vi "Icai 105.vi"() -> ()   [LabVIEW 2010]
uses:
  <vilib>/Utility/error.llb/DialogType.ctl
  <vilib>/DAQmx/write.llb/DAQmx Write (Analog DBL 1Chan 1Samp).vi
  <vilib>/DAQmx/create/channels.llb/DAQmx Create Channel (AO-Voltage-Basic).vi
  <vilib>/daqmx/miscellaneous.llb/DAQmx Fill In Error Info.vi
  <vilib>/Waveform/WDTOps.llb/WDT Append Waveforms DBL.vi
  <vilib>/measure/NI_MABase.lvlib
panel:
  out "Mod":dbl=118572.0
  out "Numeric 2":dbl=3900000.0 format="%#_7g"
  out "Numeric":dbl=3900000.0 format="%#_7g"
  in  "CAI/ICAI":bool=TRUE
  in  "DC 2":ext=3710.75 format="%.2f"
  out "?":dbl=579698.7113293351 format="%#_6f"
  in  "Fs":dbl=1000000.0
  out "#s":dbl=39524.02451426849
  in  "Time int":i32=32000
  in  "Sensitivity":u16(ring)=21 items=["2 nV/fA", "5 nV/fA", "10 nV/fA", "20 nV/fA", "50 nV/fA", "100 nV/fA", "200 nV/fA", "500 nV/fA", "1 uV/pA", "2 uV/pA", "5 uV/pA", "10 uV/pA", "20 uV/pA", "50 uV/pA", "100 uV/pA", "200 uV/pA", "500 uV/pA", "1 mV/nA", "2 mV/nA", "5 mV/nA", "10 mV/nA", "20 mV/nA", "50 mV/nA", "100 mV/nA", "200 mV/nA", "500 mV/nA", "1 V/uA"]
  in  "Detection Bandwidth":u16(ring)=7 items=["25 kHz", "8.33 kHz", "2.50 kHz", "833 Hz", "250 Hz", "83.3 Hz", "25 Hz", "8.33 Hz", "2.50 Hz", "0.833 Hz", "0.250 Hz", "0.0833 Hz", "0.025 Hz"]
  in  "SR 830 GPIB Address":i32=8
  in  "Freq 2":dbl=6401.17 format="%_7g"
  out "Iterat #":dbl=10.0
  in  "Iteration":dbl=10.0
  in  "stop 2":bool
  in  "pulse":bool=TRUE
  in  "Start":ext=0.2
  out "?":waveform(dbl)[](graph)=[{"t0"=timestamp(0 s since 1904-01-01), "dt"=1e-06, "Y"=array[3900000 elements]}, {"t0"=timestamp(0 s since 1904-01-01), "dt"=1e-06, "Y"=array[3900000 elements]}]
  in  "amplitude 2":dbl=0.25 format="%0.2p"
  in  "?":T1(ring)=enum."Triangle Wave"
  in  "phase 2":dbl format="%.2p"
  in  "Offset 2":dbl=-0.0 format="%#_6p"
  in  "frequency 4":dbl=100.0 format="%0.2p"
  in  "sampling info 4":cluster{"Fs":dbl, "#s":dbl}={"Fs"=1000000.0, "#s"=2499.0} {"Fs" format="%.2p"}
  in  "?":T1(ring)=enum."Triangle Wave"
  in  "offset 4":dbl=-1.0 format="%0.2p"
  in  "phase 4":dbl=90.0 format="%.2p"
  in  "amplitude 4":dbl=1.0 format="%0.2p"
  in  "frequency 1":dbl=100.0 format="%0.2p"
  in  "amplitude 1":dbl=1.0 format="%0.2p"
  in  "sampling info 1":cluster{"Fs":dbl, "#s":dbl}={"Fs"=1000000.0, "#s"=2500.0} {"Fs" format="%.2p"}
  in  "?":T1(ring)=enum."Triangle Wave"
  in  "phase 1":dbl=-90.0 format="%.2p"
  in  "Offset 1":dbl format="%#_6p"
  in  "iterat":dbl=2.0
  out "CW":dbl=123571.0
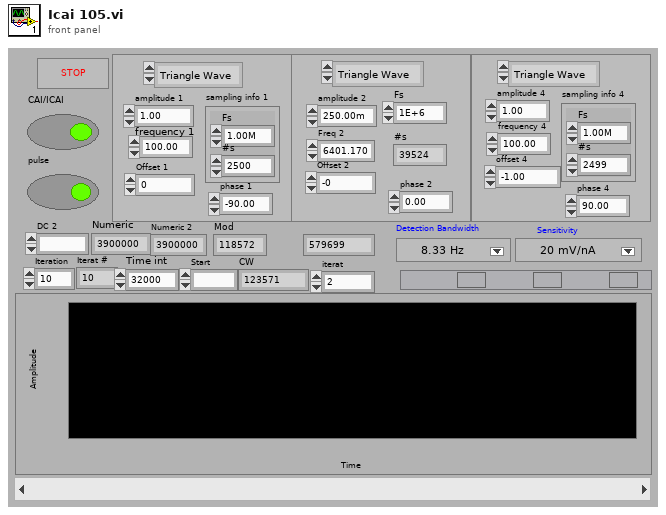
[diagram p1: front panel]
types:
  T1 = enum16{"Sine Wave", "Triangle Wave", "Square Wave", "Sawtooth Wave"}
  T2 = typedef "DialogType.ctl" = u16
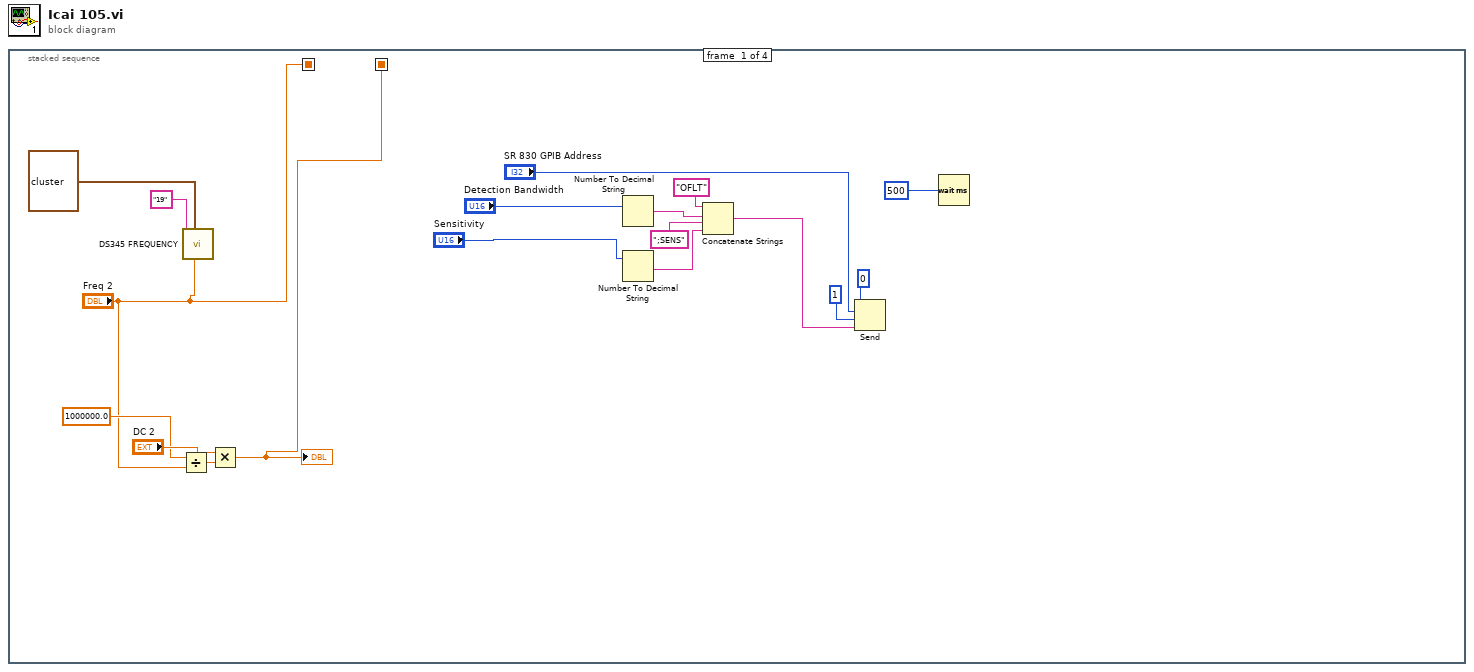
[diagram p0: block diagram]
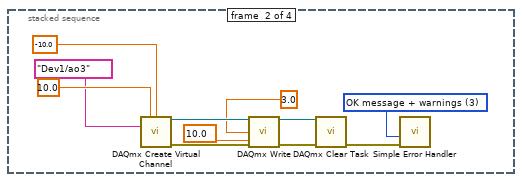
[diagram p2: hidden frame]
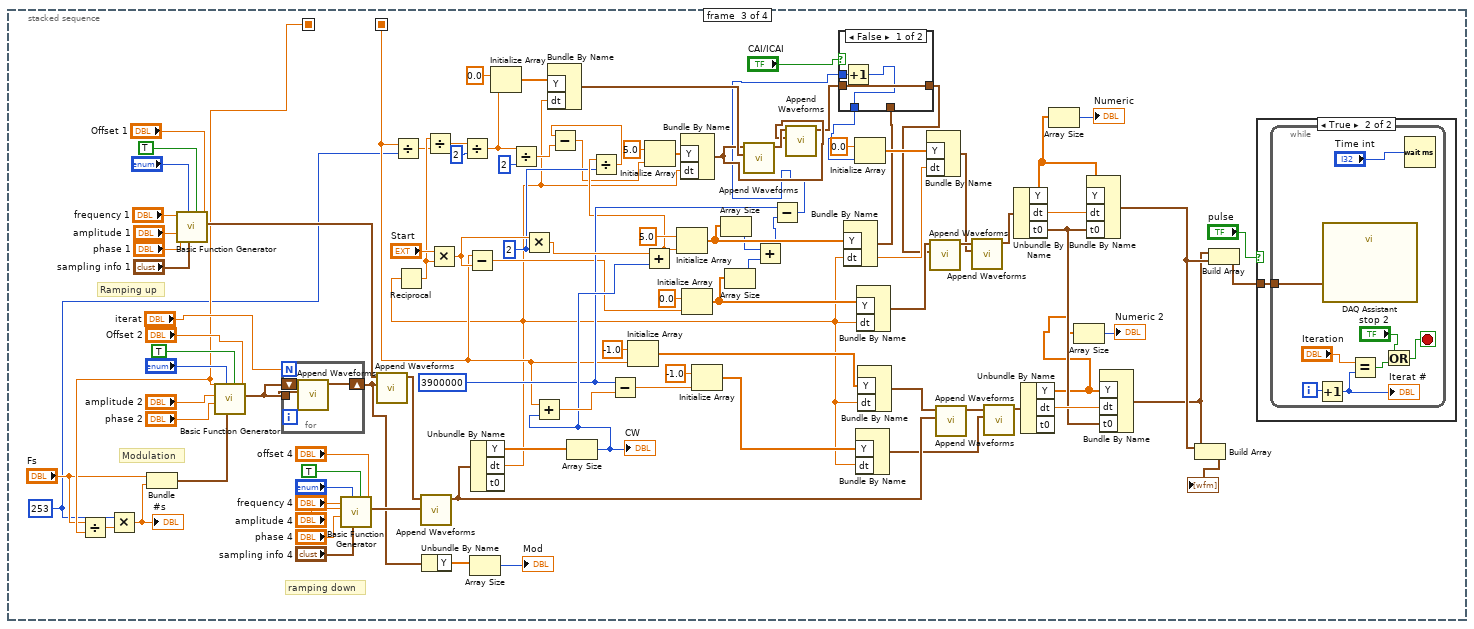
[diagram p3: hidden frame]
diagram:
  n1 = stacked-sequence {
    seq-local: ["Freq 2" _ _ _] -> [_ _ w68 _]
    seq-local: [w2 _ _ _] -> [_ _ w53 _]
    frame #0 {
      n2 = Divide(x=1000000.0 ("Fs 2"), y="Freq 2") -> (x/y=w5:dbl)
      n3 = call "DS345 FREQUENCY.vi"("GPIB address"="19", "amplitude (0 Vrms:0)"=cluster{ext, i32} {0.02, 0} ("Driving amplitude (0 Vrms:0)"), "frequency"="Freq 2") -> ()  [unwired: 5 in, 1 out]
      n4 = Multiply(x="DC 2", y=w5) -> (x*y=w2:ext)
      "?" <- w2
      n5 = Number To Decimal String(number="Detection Bandwidth") -> (decimal integer string=w15:string)  [unwired: 1 out]
      n6 = Number To Decimal String(number="Sensitivity") -> (decimal integer string=w13:string)  [unwired: 1 out]
      n7 = Concatenate Strings("OFLT", w15, ";SENS", w13) -> (w12:string)
      n8 = Send(0:0 ("bus"), 2:"SR 830 GPIB Address", 3:i16 1 ("mode"), 5:w12) -> ()  [unwired: 1 in, 3 out]
      n9 = Wait (ms)(milliseconds to wait=500) -> ()  [unwired: 1 out]
    }
    frame #1 {
      w22 = T2 3 items=["no dialog", "OK message", "continue or stop message", "OK message + warnings", "continue/stop + warnings"] ("type of dialog (OK msg:1)")
      n10 = call-poly <vilib>:"DAQmx Create Virtual Channel.vi"("maximum value"=10.0 ("Maximum Value"), "minimum value"=-10.0 ("Minimum Value"), "physical channels"=tag "Dev1/ao3" ("Physical Channel")) -> ("task out"=w25:refnum<k21>, "error out"=w26:errorcluster)  [unwired: 6 in, 5 out]
      n11 = call-poly <vilib>:"DAQmx Write.vi"("task/channels in"=w25, "data"=3.0 ("Voltage Output"), "timeout"=10.0, "error in"=w26) -> ("task out"=w20:refnum<k21>, "error out"=w21:errorcluster)  [unwired: 1 in, 9 out]
      n12 = call <vilib>:"DAQmx Clear Task.vi"("task in"=w20, "error in"=w21) -> ("error out"=w19:errorcluster)  [unwired: 13 out]
      n13 = call <vilib>:"Simple Error Handler.vi"("type of dialog (OK msg:1)"=w22, "error in (no error)"=w19) -> ()  [unwired: 8 out]
    }
    frame #2 {
      w45 = 253
      w61 = 2
      w86 = 3900000
      # "Ramping up"
      # "ramping down"
      # "Modulation"
      n14 = Divide(x="Fs", y=w68) -> (x/y=w67:dbl)
      n15 = Multiply(x=w45, y=w67) -> (x*y=w65:dbl)
      "#s" <- w65
      n16 = Bundle("Fs"="Fs", w65) -> (w64:cluster{"Fs":dbl, dbl})  [unwired: 1 out]
      n17 = call <vilib>:"Basic Function Generator.vi"("offset"="Offset 1", "reset signal"=TRUE, "sampling info"="sampling info 1", "signal type"="?", "phase"="phase 1", "amplitude"="amplitude 1", "frequency"="frequency 1") -> ("signal out"=w110:waveform(dbl))  [unwired: 2 in, 2 out]
      n18 = call <vilib>:"Basic Function Generator.vi"("offset"="Offset 2", "reset signal"=TRUE, "sampling info"=w64, "signal type"="?", "phase"="phase 2", "amplitude"="amplitude 2", "frequency"=w68) -> ("signal out"=w69:waveform(dbl))  [unwired: 2 in, 2 out]
      n19 = for {
        N: "iterat" -> [_]
        shift-right: [w148] -> w30
        shift-left: w69 -> [w146]
        tunnel: w69 -> [w147]
        n20 = call-poly <vilib>:"Append Waveforms.vi"("waveform B"=w147, "waveform A"=w146) -> ("waveform out"=w148:waveform(dbl))  [unwired: 1 in, 8 out]
      }
      n21 = call <vilib>:"Basic Function Generator.vi"("offset"="offset 4", "reset signal"=TRUE, "sampling info"="sampling info 4", "signal type"="?", "phase"="phase 4", "amplitude"="amplitude 4", "frequency"="frequency 4") -> ("signal out"=w115:waveform(dbl))  [unwired: 2 in, 2 out]
      n22 = call-poly <vilib>:"Append Waveforms.vi"("waveform B"=w30, "waveform A"=w110) -> ("waveform out"=w109:waveform(dbl))  [unwired: 1 in, 8 out]
      n23 = Divide(x=w53, y=w45) -> (x/y=w54:ext)
      n24 = call-poly <vilib>:"Append Waveforms.vi"("waveform B"=w115, "waveform A"=w109) -> ("waveform out"=w108:waveform(dbl))  [unwired: 1 in, 8 out]
      n25 = Unbundle By Name(w30) -> ("Y"=w31:dbl[])
      n26 = Array Size(array=w31) -> (size(s)=→"Mod":i32)
      n27 = Unbundle By Name(w108) -> ("Y"=w111:dbl[], "dt"=w44:dbl)  [unwired: 1 out]
      n28 = Reciprocal(x=w44) -> (1/x=w55:dbl)
      n29 = Divide(x=w55, y=w54) -> (x/y=w51:ext)
      n30 = Multiply(x="Start", y=w55) -> (x*y=w80:ext)
      n31 = Divide(x=w51, y=2) -> (x/y=w48:ext)
      n32 = Subtract(x=w53, y=w80) -> (x-y=w81:ext)
      n33 = Initialize Array(0.0 ("Trigger down"), w48) -> (w58:dbl[])
      n34 = Divide(x=w48, y=2) -> (x/y=w46:ext)
      n35 = Multiply(x=w80, y=w61) -> (x*y=w88:ext)
      n36 = Bundle By Name("Y"=w58, "dt"=w44) -> (w57:waveform(dbl))  [unwired: 1 out]
      n37 = Array Size(array=w111) -> (size(s)=w87:i32)
      "CW" <- w87
      n38 = Add(x=w53, y=w87) -> (x+y=w92:ext)
      n39 = Subtract(x=w86, y=w92) -> (x-y=w91:ext)
      n40 = Initialize Array(-1.0 ("DC level"), w53) -> (w94:dbl[])
      n41 = Add(x=w88, y=w87) -> (x+y=w62:ext)
      n42 = Divide(x=w62, y=w61) -> (x/y=w50:ext)
      n43 = Subtract(x=w50, y=w46) -> (x-y=w49:ext)
      n44 = Initialize Array(5.0 ("Trigger up"), w49) -> (w60:dbl[])
      n45 = Initialize Array(5.0 ("Trigger up"), w62) -> (w78:dbl[])
      n46 = Bundle By Name("Y"=w60, "dt"=w44) -> (w43:waveform(dbl))  [unwired: 1 out]
      n47 = Initialize Array(0.0 ("Trigger down"), w81) -> (w79:dbl[])
      n48 = Initialize Array(-1.0 ("DC level"), w91) -> (w90:dbl[])
      n49 = Array Size(array=w78) -> (size(s)=w76:i32)
      n50 = Array Size(array=w79) -> (size(s)=w77:i32)
      n51 = call-poly <vilib>:"Append Waveforms.vi"("waveform B"=w57, "waveform A"=w43) -> ("waveform out"=w56:waveform(dbl))  [unwired: 1 in, 8 out]
      n52 = Add(x=w76, y=w77) -> (x+y=w75:i32)
      n53 = Subtract(x=w86, y=w75) -> (x-y=w34:i32)
      n54 = call-poly <vilib>:"Append Waveforms.vi"("waveform B"=w43, "waveform A"=w56) -> ("waveform out"=w42:waveform(dbl))  [unwired: 1 in, 8 out]
      n55 = Bundle By Name("Y"=w78, "dt"=w44) -> (w40:waveform(dbl))  [unwired: 1 out]
      n56 = case shown="False" "CAI/ICAI" {
        tunnel: w42 -> [w134 _]
        tunnel: [w134 w136] -> w41
        tunnel: w40 -> [_ w136]
        tunnel: w34 -> [w133 w135]
        tunnel: [w132 w135] -> w33
        frame False {
          n57 = Increment(x=w133) -> (x+1=w132:i32)
        }
        frame True {
        }
      }
      n58 = Initialize Array(0.0 ("Trigger down"), w33) -> (w84:dbl[])
      n59 = Bundle By Name("Y"=w90, "dt"=w44) -> (w89:waveform(dbl))  [unwired: 1 out]
      n60 = Bundle By Name("Y"=w79, "dt"=w44) -> (w83:waveform(dbl))  [unwired: 1 out]
      n61 = Bundle By Name("Y"=w94, "dt"=w44) -> (w113:waveform(dbl))  [unwired: 1 out]
      n62 = Bundle By Name("Y"=w84, "dt"=w44) -> (w82:waveform(dbl))  [unwired: 1 out]
      n63 = call-poly <vilib>:"Append Waveforms.vi"("waveform B"=w41, "waveform A"=w83) -> ("waveform out"=w105:waveform(dbl))  [unwired: 1 in, 8 out]
      n64 = call-poly <vilib>:"Append Waveforms.vi"("waveform B"=w108, "waveform A"=w113) -> ("waveform out"=w114:waveform(dbl))  [unwired: 1 in, 8 out]
      n65 = call-poly <vilib>:"Append Waveforms.vi"("waveform B"=w82, "waveform A"=w105) -> ("waveform out"=w101:waveform(dbl))  [unwired: 1 in, 8 out]
      n66 = call-poly <vilib>:"Append Waveforms.vi"("waveform B"=w89, "waveform A"=w114) -> ("waveform out"=w98:waveform(dbl))  [unwired: 1 in, 8 out]
      n67 = Unbundle By Name(w101) -> ("Y"=w37:dbl[], "dt"=w100:dbl, "t0"=w74:timestamp)
      n68 = Unbundle By Name(w98) -> ("Y"=w35:dbl[], "dt"=w97:dbl)  [unwired: 1 out]
      n69 = Array Size(array=w37) -> (size(s)=→"Numeric":i32)
      n70 = Array Size(array=w35) -> (size(s)=→"Numeric 2":i32)
      n71 = Bundle By Name("Y"=w37, "dt"=w100, "t0"=w74) -> (w99:waveform(dbl))  [unwired: 1 out]
      n72 = Bundle By Name("Y"=w35, "dt"=w97, "t0"=w74) -> (w96:waveform(dbl))  [unwired: 1 out]
      n73 = Build Array(w99, w96) -> (→"?":waveform(dbl)[])
      n74 = Build Array(w96, w99) -> (w102:waveform(dbl)[])
      n75 = case shown="True" "pulse" {
        tunnel: w102 -> [_ w137]
        frame False {
        }
        frame True {
          n76 = while {
            tunnel: w137 -> [w138]
            i -> [w142]
            stop <- w143 stop-if-true
            n77 = Increment(x=w142) -> (x+1=w140:i32)
            "Iterat #" <- w140
            n78 = call "DAQ Assistant"("data"=w138) -> ()  [unwired: 3 in, 16 out]
            n79 = Equal?(x="Iteration", y=w140) -> (x = y?=w145:bool)
            n80 = Or(x="stop 2", y=w145) -> (x .or. y?=w143:bool)
            n81 = Wait (ms)(milliseconds to wait="Time int") -> ()  [unwired: 1 out]
          }
        }
      }
    }
    frame #3 {
    }
  }
